vi "setGlobalData.vi"   [LabVIEW 2014]
uses:
  Robot Global Data.vi
  <vilib>/Rock Robotics/Network Tables/SD Write Boolean.vi
types:
  T1 = typedef "WPI_SwitchDevRef.ctl" = cluster{"DevStatus":errorcluster, "DIO Channel":T2, "Controller":T3, "CntIndex":T4, "Normally Closed":bool}
  T2 = typedef "FPGA_DIOChannel.ctl" = enum8{"DIO 0", "DIO 1", "DIO 2", "DIO 3", "DIO 4", "DIO 5", "DIO 6", "DIO 7", "DIO 8", "DIO 9", "DIO MXP 0", "DIO MXP 1", "DIO MXP 2", "DIO MXP 3", "DIO MXP 4", "DIO MXP 5", "DIO MXP 6", "DIO MXP 7", "DIO MXP 8", "DIO MXP 9", "DIO MXP 10", "DIO MXP 11", "DIO MXP 12", "DIO MXP 13", "DIO MXP 14", "DIO MXP 15", "Invalid"}
  T3 = typedef "FPGA_TypedefDigitalModule.ctl" = enum16{"Controller 1"}
  T4 = typedef "FPGA_CounterCtrSystemIndex.ctl" = enum8{"Ctr 0", "Ctr 1", "Ctr 2", "Ctr 3", "Ctr 4", "Ctr 5", "Ctr 6", "Ctr 7", "Invalid"}
  T5 = typedef "WPI_EncoderDevRef.ctl" = cluster{"DevStatus":errorcluster, "EncoderIndex":T6, "CounterIndex":T4, "DistancePerCount":dbl, "Decoding Type":T7}
  T6 = typedef "FPGA_EncoderIdx.ctl" = enum8{"Enc 0", "Enc 1", "Enc 2", "Enc 3", "Enc 4", "Enc 5", "Enc 6", "Enc 7", "Invalid"}
  T7 = typedef "WPI_EncoderType.ctl" = enum16{"1x", "2x", "4x"}
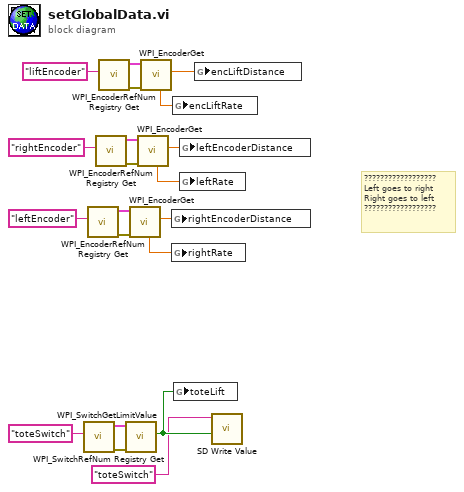
[diagram p0: block diagram]
diagram:
  # "??????????????????\nLeft goes to right\nRight goes to left\n??????????????????"
  n1 = call <vilib>:"WPI_SwitchRefNum Registry Get.vi"("refnum name"="toteSwitch") -> ("error out"=w10:errorcluster, "SwitchDevRef"=w9:T1)  [unwired: 9 in]
  n2 = call <vilib>:"WPI_EncoderRefNum Registry Get.vi"("refnum name"="leftEncoder") -> ("error out"=w20:errorcluster, "EncoderDevRef"=w19:T5)  [unwired: 9 in]
  n3 = call <vilib>:"WPI_EncoderRefNum Registry Get.vi"("refnum name"="rightEncoder") -> ("error out"=w15:errorcluster, "EncoderDevRef"=w16:T5)  [unwired: 9 in]
  n4 = call <vilib>:"WPI_EncoderRefNum Registry Get.vi"("refnum name"="liftEncoder") -> ("error out"=w3:errorcluster, "EncoderDevRef"=w2:T5)  [unwired: 9 in]
  n5 = call <vilib>:"WPI_SwitchGetLimitValue.vi"("error in (no error)"=w10, "SwitchDevRef"=w9) -> ("Switch Pressed"=w7:bool)  [unwired: 7 in, 2 out]
  n6 = call <vilib>:"WPI_EncoderGet.vi"("error in (no error)"=w20, "EncoderDevRef"=w19) -> ("Distance"=w12:dbl, "Rate"=w11:dbl)  [unwired: 4 in, 4 out]
  n7 = call <vilib>:"WPI_EncoderGet.vi"("error in (no error)"=w15, "EncoderDevRef"=w16) -> ("Distance"=w13:dbl, "Rate"=w14:dbl)  [unwired: 4 in, 4 out]
  n8 = call <vilib>:"WPI_EncoderGet.vi"("error in (no error)"=w3, "EncoderDevRef"=w2) -> ("Distance"=w5:dbl, "Rate"=w4:dbl)  [unwired: 4 in, 4 out]
  n9 = global write "Robot Global Data.vi" "rightEncoderDistance"(w12) -> ()
  n10 = global write "Robot Global Data.vi" "rightRate"(w11) -> ()
  n11 = global write "Robot Global Data.vi" "encLiftRate"(w4) -> ()
  n12 = global write "Robot Global Data.vi" "toteLift"(w7) -> ()
  n13 = global write "Robot Global Data.vi" "leftEncoderDistance"(w13) -> ()
  n14 = global write "Robot Global Data.vi" "leftRate"(w14) -> ()
  n15 = global write "Robot Global Data.vi" "encLiftDistance"(w5) -> ()
  n16 = call-poly <vilib>:"SD Write Value.vi"("Boolean"=w7, "Name"="toteSwitch") -> ()  [unwired: 8 in, 2 out]
